vi "MecaDrivePoseEst2_InterpRecord_ExtractFromVar.vi"(11 "OutputVariant":variant) -> (0 "error out":errorcluster, 3 "out InterpRecord":T1={"PoseMeters"={"TRANSLATION"={"X"=0.0, "Y"=0.0}, "ROTATION"={"VALUE"=0.0, "COS"=1.0, "SIN"=0.0}}, "GyroAngle"={"VALUE"=0.0, "COS"=1.0, "SIN"=0.0}, "ModulePositions"={"FrontLeft"=0.0, "FrontRight"=0.0, "RearLeft"=0.0, "RearRight"=0.0, "P"=FALSE}} {"ModulePositions"."RearRight" format="%19.3f"; "ModulePositions"."RearLeft" format="%19.3f"; "ModulePositions"."FrontRight" format="%19.3f"; "ModulePositions"."FrontLeft" format="%19.3f"; "GyroAngle"."SIN" format="%13.4f"; "GyroAngle"."COS" format="%13.4f"; "GyroAngle"."VALUE" format="%13.4f"; "PoseMeters"."ROTATION"."SIN" format="%13.4f"; "PoseMeters"."ROTATION"."COS" format="%13.4f"; "PoseMeters"."ROTATION"."VALUE" format="%13.4f"; "PoseMeters"."TRANSLATION"."Y" format="%14.3f"; "PoseMeters"."TRANSLATION"."X" format="%14.3f"})   [LabVIEW 2019, in "Trajectory_Library.lvlib"]
doc: "This extracts the specific data cluster of Swerve Drive Pose Estimator2 Interpolation Record from a Variant.\n\nThis is an internal routine. It should NOT be called by the end user."
uses:
  Trajectory_Library.lvlib
  TypeDef/MECA_DRIVE_POSE_EST2_INTERP_RECORD.ctl
  TypeDef/POSE2D.ctl
  TypeDef/TRANSLATION2D.ctl
  TypeDef/ROTATION2D.ctl
  TypeDef/MECA_WHEEL_POSITIONS.ctl
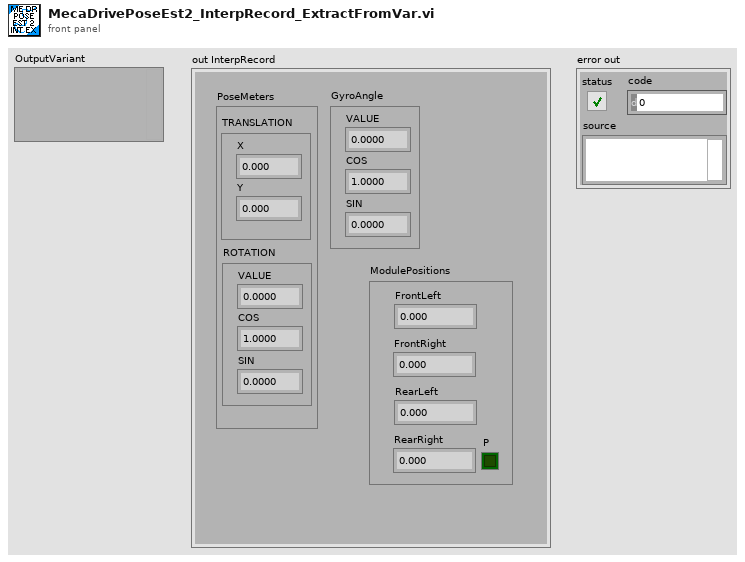
[diagram p1: front panel]
types:
  T1 = typedef "Trajectory_Library.lvlib/MECA_DRIVE_POSE_EST2_INTERP_RECORD.ctl" = cluster{"PoseMeters":T2, "GyroAngle":T4, "ModulePositions":T5}
  T2 = typedef "Trajectory_Library.lvlib/POSE2D.ctl" = cluster{"TRANSLATION":T3, "ROTATION":T4}
  T3 = typedef "Trajectory_Library.lvlib/TRANSLATION2D.ctl" = cluster{"X":dbl, "Y":dbl}
  T4 = typedef "Trajectory_Library.lvlib/ROTATION2D.ctl" = cluster{"VALUE":dbl, "COS":dbl, "SIN":dbl}
  T5 = typedef "Trajectory_Library.lvlib/MECA_WHEEL_POSITIONS.ctl" = cluster{"FrontLeft":dbl, "FrontRight":dbl, "RearLeft":dbl, "RearRight":dbl, "P":bool}
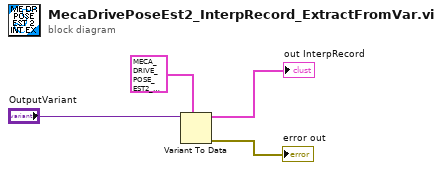
[diagram p0: block diagram]
diagram:
  n1 = Variant To Data(type=T1 {"PoseMeters"={"TRANSLATION"={"X"=0.0, "Y"=0.0}, "ROTATION"={"VALUE"=0.0, "COS"=1.0, "SIN"=0.0}}, "GyroAngle"={"VALUE"=0.0, "COS"=1.0, "SIN"=0.0}, "ModulePositions"={"FrontLeft"=0.0, "FrontRight"=0.0, "RearLeft"=0.0, "RearRight"=0.0, "P"=FALSE}} ("MECA_DRIVE_POSE_EST2_INTERP_RECORD"), Variant="OutputVariant") -> (data=→"out InterpRecord":T1, error out=→"error out":errorcluster)  [unwired: 1 in]
